vi "AB_Set_Source_Property.vi"(8 "error in (no error)":errorcluster, 9 "property value":variant, 10 "property name":T1, 11 "Source in":refnum<class "AB_Source.lvclass">) -> (0 "error out":errorcluster, 3 "Source out":refnum<class "AB_Source.lvclass">)   [LabVIEW 2020]
uses:
  <vilib>/AppBuilder/AB_Classes/Source/AB_Source.lvclass
  <vilib>/AppBuilder/AB_Source_Property_Type.ctl
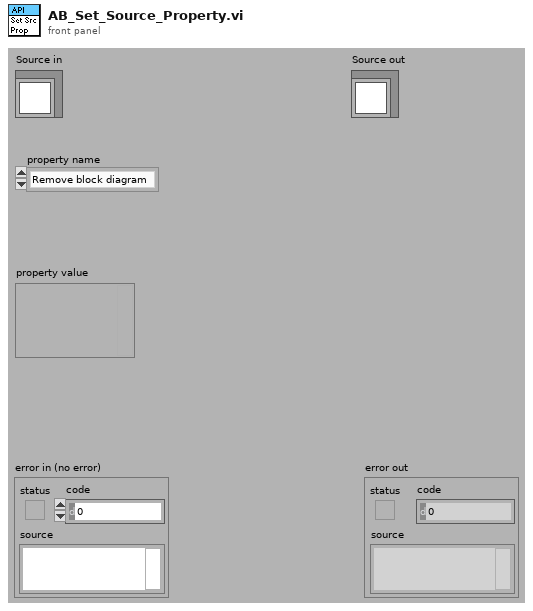
[diagram p1: front panel]
types:
  T1 = typedef "AB_Source_Property_Type.ctl" = enum16{"Remove block diagram", "Remove front panel", "Password", "Window has title bar", "Show menu bar", "Show vertical scroll bar", "Show horizontal scroll bar", "Show toolbar", "Show Abort button", "Show fp when called", "Window behavior", "Allow user to close window", "Window run-time position", "Run when opened", "Allow debugging", "Auto error handling", "Generate guard code", "Use stack variables", "Expression folding", "Integer only", "Inline subVI"}
  T2 = typedef "AB_Source.ctl" = cluster{"path":path, "itemID":string, "parentIndex":i32, "sourceInclusion":T3, "destinationIndex":i32, "properties":T4[], "newName":string, "lvfile":bool, "valid":bool, "eng_inBuild":bool, "eng_isNonVILink":bool, "Amalgamation":bool, "Amalgamation Piece":bool, "eng_delimitedName":string, "preventRename":bool}
  T3 = typedef "AB_Source_Inclusion.ctl" = enum16{"IncludeIfReferenced", "Include", "Exclude", "TopLevel"}
  T4 = typedef "AB_Source_Properties.ctl" = cluster{"sourcePropertyType":T1, "value":variant}
  T5 = cluster{"property name":T1, "property value":variant}
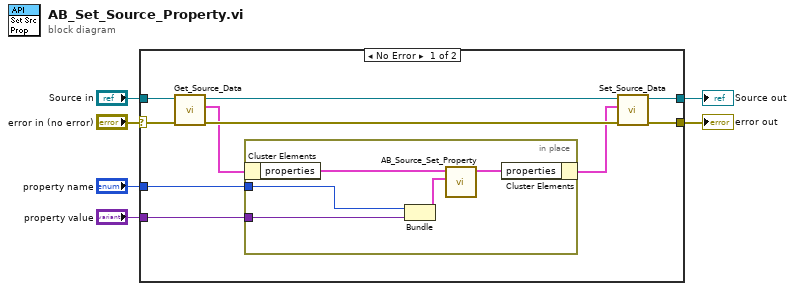
[diagram p0: block diagram]
diagram:
  n1 = case shown="No Error" "error in (no error)" {
    selector: "error in (no error)" -> [w8 w23]
    tunnel: [w7 w23] -> w5
    tunnel: [w12 w22] -> w4
    tunnel: "Source in" -> [w11 w22]
    tunnel: "property name" -> [w10 _]
    tunnel: "property value" -> [w9 _]
    frame No Error {
      n2 = call <vilib>:"Get_Source_Data.vi"("error in (no error)"=w8, "Class in"=w11) -> ("error out"=w15:errorcluster, "data"=w14:T2, "Class out"=w16:refnum<class "AB_Source.lvclass">)  [unwired: 7 out]
      n3 = in-place {
        in-place-border: w10 -> [w18]
        in-place-border: w9 -> [w17]
        n4 = in-place-cluster #1(w14) -> ("properties"=w20:T4[])
        n5 = Bundle("property name"=w18, "property value"=w17) -> (w21:T5)  [unwired: 1 out]
        n6 = call <vilib>:"AB_Source_Set_Property.vi"("sourceProperty"=w21, "sourceProperties in"=w20) -> ("sourceProperties out"=w19:T4[])  [unwired: 1 in, 8 out]
        n7 = in-place-cluster #1("properties"=w19) -> (w13:T2)
      }
      n8 = call <vilib>:"Set_Source_Data.vi"("error in (no error)"=w15, "data"=w13, "Class in"=w16) -> ("error out"=w7:errorcluster, "Class out"=w12:refnum<class "AB_Source.lvclass">)  [unwired: 7 out]
    }
    frame Error {
    }
  }
  "error out" <- w5
  "Source out" <- w4
